vi "SlotBoolGV.vi"(6 "Slot":T3, 9 "Para":T2={"Action"=enum."Set", "GVName"=enum."SlotStop"}, 10 "Bool":bool) -> (2 "Value":bool)   [LabVIEW 2013]
uses:
  SysControl/Slot.ctl
  SysControl/SlotGV.ctl
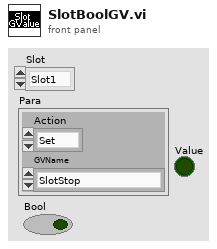
[diagram p1: front panel]
types:
  T1 = typedef "SlotGV.ctl" = enum16{"SlotReady", "SNReady", "SlotStart", "SlotStop"}
  T2 = cluster{"Action":enum16{"Get", "Set", "Init"}, "GVName":T1}
  T3 = typedef "Slot.ctl" = enum16{"Slot1", "Slot2", "Slot3", "Slot4"}
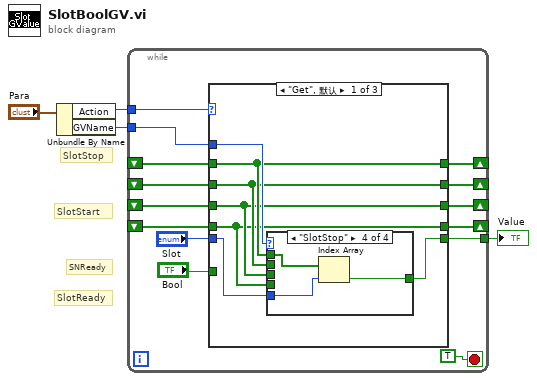
[diagram p0: block diagram]
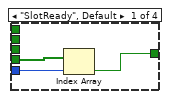
[diagram p2: hidden frame]
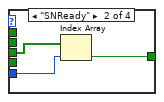
[diagram p3: hidden frame]
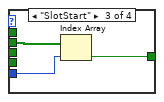
[diagram p4: hidden frame]
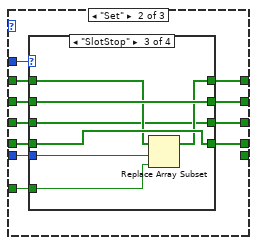
[diagram p5: hidden frame]
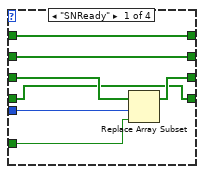
[diagram p6: hidden frame]
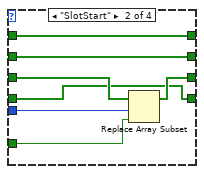
[diagram p7: hidden frame]
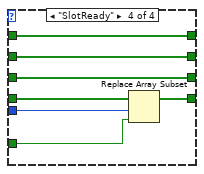
[diagram p8: hidden frame]
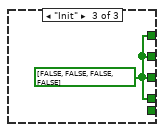
[diagram p9: hidden frame]
diagram:
  # "SlotStop"
  # "SlotStart"
  # "SNReady"
  # "SlotReady"
  n1 = Unbundle By Name("Para") -> ("Action"=w2:enum16{"Get", "Set", "Init"}, "GVName"=w1:T1)
  n2 = while {
    shift-right: [w16] -> _
    shift-left: _ -> [w17]
    shift-right: [w15] -> _
    shift-left: _ -> [w12]
    shift-right: [w14] -> _
    shift-left: _ -> [w11]
    shift-right: [w13] -> _
    shift-left: _ -> [w10]
    tunnel: [w8] -> w4
    tunnel: w2 -> [w6]
    tunnel: w1 -> [w5]
    stop <- TRUE stop-if-true
    n3 = case shown="\"Get\", 默认" w6 {
      tunnel: w17 -> [w24 w48 _]
      tunnel: [w24 w47 w77] -> w16
      tunnel: "Slot" -> [w23 w46 _]
      tunnel: [w21 w40 w77] -> w15
      tunnel: [w20 w39 w77] -> w14
      tunnel: [w19 w43 w77] -> w13
      tunnel: w5 -> [w25 w45 _]
      tunnel: w12 -> [w21 w42 _]
      tunnel: w11 -> [w20 w41 _]
      tunnel: w10 -> [w19 w44 _]
      tunnel: "Bool" -> [_ w38 _]
      tunnel: [w22 _ _] -> w8
      frame "Get", Default {
        n4 = case shown="\"SlotStop\"" w25 {
          tunnel: w19 -> [w28 _ _ _]
          tunnel: w20 -> [_ w29 _ _]
          tunnel: w21 -> [_ _ w32 _]
          tunnel: w24 -> [_ _ _ w35]
          tunnel: w23 -> [w27 w31 w34 w37]
          tunnel: [w26 w30 w33 w36] -> w22
          frame "SlotReady", Default {
            n5 = Index Array(array=w28, index=w27) -> (element=w26:bool)
          }
          frame "SNReady" {
            n6 = Index Array(array=w29, index=w31) -> (element=w30:bool)
          }
          frame "SlotStart" {
            n7 = Index Array(array=w32, index=w34) -> (element=w33:bool)
          }
          frame "SlotStop" {
            n8 = Index Array(array=w35, index=w37) -> (element=w36:bool)
          }
        }
      }
      frame "Set" {
        n9 = case shown="\"SlotStop\"" w45 {
          tunnel: w48 -> [w54 w61 w64 w70]
          tunnel: [w54 w61 w65 w70] -> w47
          tunnel: w46 -> [w55 w62 w69 w76]
          tunnel: w44 -> [w49 w56 w66 w72]
          tunnel: [w49 w56 w66 w71] -> w43
          tunnel: w42 -> [w53 w60 w68 w75]
          tunnel: w41 -> [w51 w58 w63 w73]
          tunnel: [w50 w57 w63 w73] -> w39
          tunnel: [w53 w60 w68 w75] -> w40
          tunnel: w38 -> [w52 w59 w67 w74]
          frame "SNReady" {
            n10 = Replace Array Subset(array=w51, new element=w52, index=w55) -> (w50:bool[])
          }
          frame "SlotStart" {
            n11 = Replace Array Subset(array=w58, new element=w59, index=w62) -> (w57:bool[])
          }
          frame "SlotStop" {
            n12 = Replace Array Subset(array=w64, new element=w67, index=w69) -> (w65:bool[])
          }
          frame "SlotReady" {
            n13 = Replace Array Subset(array=w72, new element=w74, index=w76) -> (w71:bool[])
          }
        }
      }
      frame "Init" {
        w77 = bool[] [FALSE, FALSE, FALSE, FALSE] ("ArrayIn")
      }
    }
  }
  "Value" <- w4
